vi "testError.vi"(8 "error in (no error)":errorcluster) -> (0 "error out":errorcluster)   [LabVIEW 2019, in "AssertionTest.lvlib" / "AssertTrue.lvlib"]
uses:
  AssertTrue.lvlib
  <vilib>/Utility/error.llb/Error Cluster From Error Code.vi
  <vilib>/ErrorRing/Error Ring.xnode
  Assertion/Assertion.lvlib
  AssertionTest.lvlib
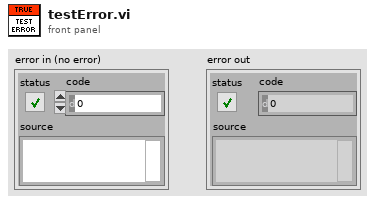
[diagram p1: front panel]
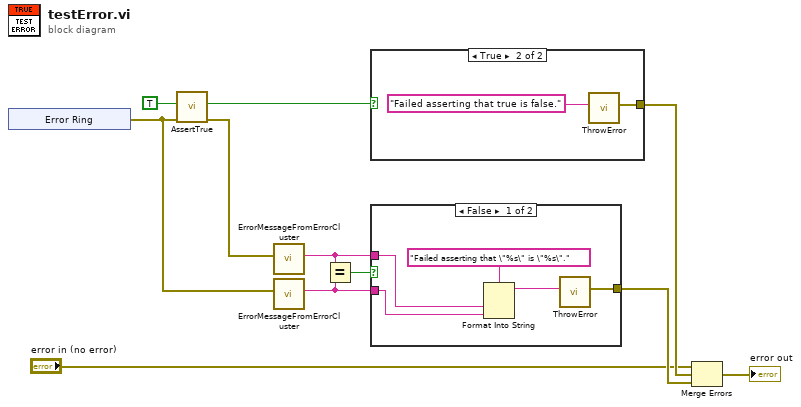
[diagram p0: block diagram]
diagram:
  n1 = xnode "Error Ring"() -> ("error out"=w8:errorcluster)
  n2 = call "AssertTrue.vi"("error in (no error)"=w8, "Condition"=TRUE) -> ("error out"=w10:errorcluster, "Result"=w9:bool)  [unwired: 8 in]
  n3 = call "ErrorMessageFromErrorCluster.vi"("Error"=w10) -> ("Error Message"=w6:string)  [unwired: 10 in]
  n4 = call "ErrorMessageFromErrorCluster.vi"("Error"=w8) -> ("Error Message"=w5:string)  [unwired: 10 in]
  n5 = Equal?(x=w6, y=w5) -> (x = y?=w7:bool)
  n6 = case shown="True" w9 {
    tunnel: [_ w12] -> w3
    frame False {
    }
    frame True {
      n7 = call "ThrowError.vi"("Error Message"="Failed asserting that true is false." ("message")) -> ("error out"=w12:errorcluster)  [unwired: 10 in]
    }
  }
  n8 = case shown="False" w7 {
    tunnel: w6 -> [w17 _]
    tunnel: w5 -> [w16 _]
    tunnel: [w14 _] -> w4
    frame False {
      n9 = Format Into String(format string="Failed asserting that \"%s\" is \"%s\".", w17, w16) -> (resulting string=w15:string)  [unwired: 2 in, 1 out]
      n10 = call "ThrowError.vi"("Error Message"=w15) -> ("error out"=w14:errorcluster)  [unwired: 10 in]
    }
    frame True {
    }
  }
  n11 = Merge Errors("error in (no error)", w3, w4) -> (→"error out":errorcluster)
